vi "GetFirstScreen.vi"(8 "error in (no error)":errorcluster, 11 "Pong in":refnum<class "Pong.lvclass">) -> (0 "error out":errorcluster, 2 "Array":u32[][](array[numeric]), 3 "Pong out":refnum<class "Pong.lvclass">)   [LabVIEW 2019, in "RT_Game.lvlib" / "Pong.lvclass"]
uses:
  Pong.lvclass
  Game/Game.lvclass
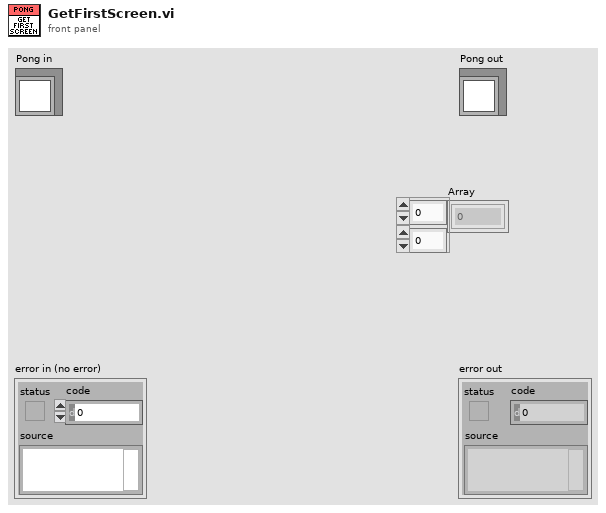
[diagram p1: front panel]
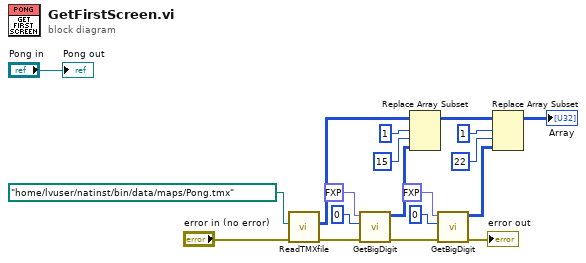
[diagram p0: block diagram]
diagram:
  n1 = call "ReadTMXfile.vi"("error in (no error)"="error in (no error)", "path to tmx-file (created with Tiles2D)"=path "/home/lvuser/natinst/bin/data/maps/Pong.tmx") -> ("error out"=w17:errorcluster, "Tilenumbers"=w15:u32[][])  [unwired: 8 in]
  n2 = call "GetBigDigit.vi"("error in (no error)"=w17, "Digit"=0, "color"=fxp<+,3,3> 1.0) -> ("error out"=w14:errorcluster, "Array"=w8:u32[][])  [unwired: 7 in]
  n3 = Replace Array Subset(array=w15, new element=w8, index (row)=1, index (col)=15 ("disabled index (col)")) -> (w11:u32[][])
  n4 = call "GetBigDigit.vi"("error in (no error)"=w14, "Digit"=0, "color"=fxp<+,3,3> 2.0) -> ("error out"=→"error out":errorcluster, "Array"=w1:u32[][])  [unwired: 7 in]
  n5 = Replace Array Subset(array=w11, new element=w1, index (row)=1, index (col)=22 ("disabled index (col)")) -> (→"Array":u32[][])
  "Pong out" <- "Pong in"
